vi "BRig_dataAnalog_valueAI1_3.vi"() -> (2 "output_valueAI1_3":i32)   [LabVIEW 2014]
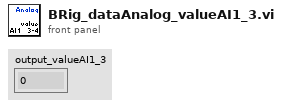
[diagram p1: front panel]
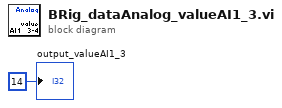
[diagram p0: block diagram]
diagram:
  "output_valueAI1_3" <- 14 ("output_iBlock")
